vi "Status Msg Q DVR.vi"(10 "Msg Q DVR":refnum<data-value>) -> (0 "error out":errorcluster, 2 "Msg Q DVR Alias":string)   [LabVIEW 2021, in "LVCAM.lvlib" / "Actor.lvclass"]
uses:
  Actor.lvclass
  Msg/Msg.lvclass
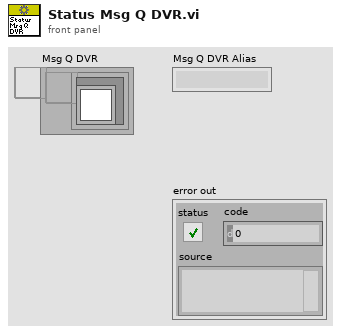
[diagram p1: front panel]
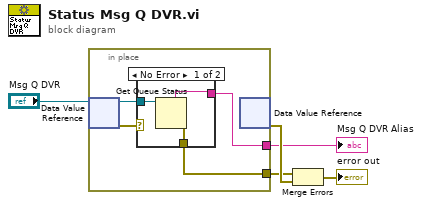
[diagram p0: block diagram]
diagram:
  n1 = in-place {
    in-place-border: [w8] -> w1
    in-place-border: [w7] -> w2
    n2 = in-place-dvr #1("Msg Q DVR") -> (w9:refnum<queue>, w6:errorcluster)
    n3 = case shown="No Error" w6 {
      selector: w6 -> [_ w13]
      tunnel: w9 -> [w12 _]
      tunnel: [w11 w13] -> w8
      tunnel: [w10 _] -> w7
      frame No Error {
        n4 = Get Queue Status(queue=w12) -> (queue name=w10:string, error out=w11:errorcluster)  [unwired: 2 in, 6 out]
      }
      frame Error {
      }
    }
    n5 = in-place-dvr #1() -> (w3:errorcluster)  [unwired: 1 in, 1 out]
  }
  "Msg Q DVR Alias" <- w2
  n6 = Merge Errors(w1, w3) -> (→"error out":errorcluster)
